vi "sub_average_amplitude.vi"(11 "Input CSI sample":cdb[][][](array[numeric])) -> (3 "Array":dbl[](array[numeric]))   [LabVIEW 2020]
uses:
  <vilib>/Analysis/baseanly.llb/Mean (DBL).vi
  <vilib>/Analysis/NI_AALBase.lvlib
panel:
  out "size(s)":i32[](array[numeric])
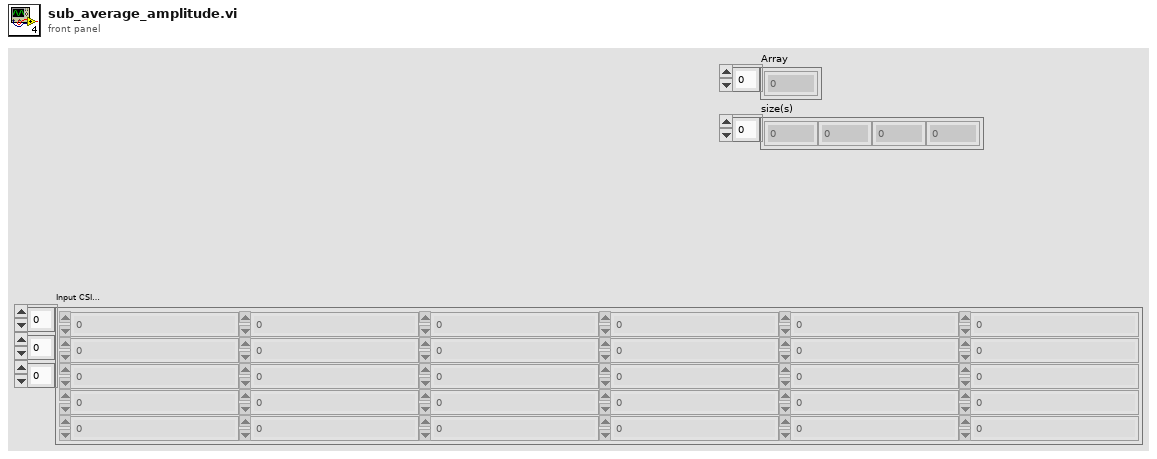
[diagram p1: front panel]
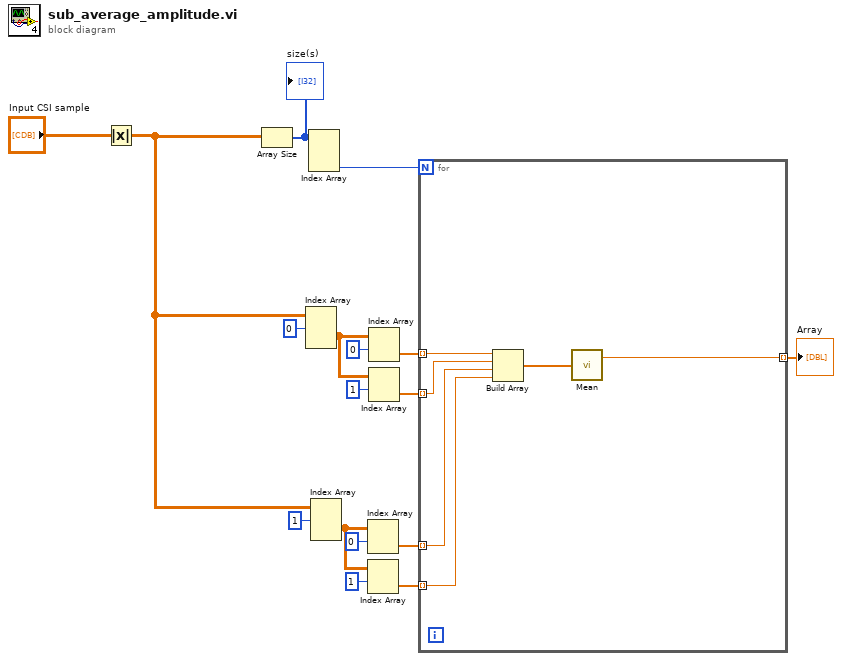
[diagram p0: block diagram]
diagram:
  n1 = Absolute Value ("Absolute Value.vi")(x="Input CSI sample") -> (abs(x)=w2:dbl[][][])
  n2 = Array Size(array=w2) -> (size(s)=w17:i32[])
  "size(s)" <- w17
  n3 = Index Array(array=w2, index (dim 0)=0 ("index (page)")) -> (element=w12:dbl[][])  [unwired: 2 in]
  n4 = Index Array(array=w17) -> (element #3=w16:i32)  [unwired: 3 in, 2 out]
  n5 = Index Array(array=w2, index (dim 0)=1 ("index (page)")) -> (element=w10:dbl[][])  [unwired: 2 in]
  n6 = Index Array(array=w10, index (row)=0) -> (element=w5:dbl[])  [unwired: 1 in]
  n7 = Index Array(array=w10, index (row)=1) -> (element=w4:dbl[])  [unwired: 1 in]
  n8 = Index Array(array=w12, index (row)=0) -> (element=w7:dbl[])  [unwired: 1 in]
  n9 = Index Array(array=w12, index (row)=1) -> (element=w6:dbl[])  [unwired: 1 in]
  n10 = for {
    N: w16 -> [_]
    tunnel: w7 -> [w23] mode=indexing
    tunnel: w6 -> [w22] mode=indexing
    tunnel: w5 -> [w21] mode=indexing
    tunnel: w4 -> [w20] mode=indexing
    tunnel: [w18] -> w1 mode=indexing
    n11 = Build Array(w23, w22, w21, w20) -> (w19:dbl[])
    n12 = call-poly <vilib>:"Mean.vi"("X"=w19) -> ("mean"=w18:dbl)  [unwired: 1 out]
  }
  "Array" <- w1
